vi "Open.vi"(8 "error in (no error)":errorcluster caption="entrée d'erreur (pas d'erreur)", 11 "Path In":path) -> (0 "error out":errorcluster caption="sortie d'erreur", 3 "Open Out":string)   [LabVIEW 2012, in "TiffLib_v1.lvlib"]
uses:
  TiffLib_v1.lvlib
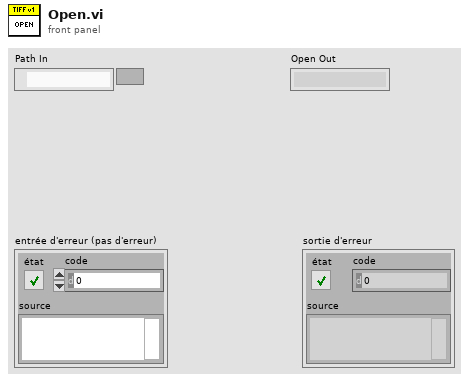
[diagram p1: front panel]
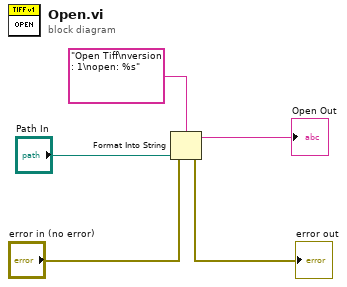
[diagram p0: block diagram]
diagram:
  n1 = Format Into String(format string="Open Tiff\nversion : 1\nopen: %s" ("chaîne de format"), error in="error in (no error)", "Path In") -> (resulting string=→"Open Out":string, error out=→"error out":errorcluster)  [unwired: 1 in]
